vi "DEV scaler to LV Array Issue 67.vi"() -> ()   [LabVIEW 2017]
uses:
  JSONtext.lvlib
panel:
  out "data":cluster{"A":string[], "B":dbl[]}
  out "Variant out":variant
  out "error out":errorcluster
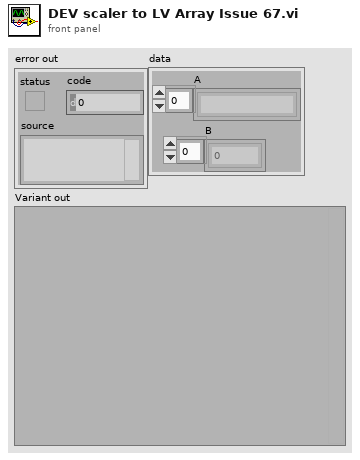
[diagram p1: front panel]
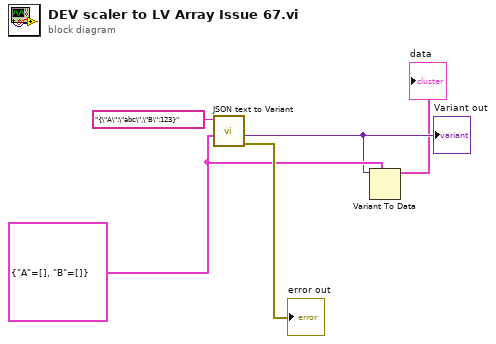
[diagram p0: block diagram]
diagram:
  w3 = cluster{"A":string[], "B":dbl[]} {"A"=[], "B"=[]}
  n1 = call "JSON text to Variant.vi"("Data Type"=w3, "JSON"="{\"A\":\"abc\",\"B\":123}") -> ("error out"=→"error out":errorcluster, "Variant out"=w2:variant)  [unwired: 8 in]
  "Variant out" <- w2
  n2 = Variant To Data(type=w3, Variant=w2) -> (data=→"data":cluster{"A":string[], "B":dbl[]})  [unwired: 1 in, 1 out]
